vi "Delete.vi"() -> ()   [LabVIEW 2020]
uses:
  <vilib>/httpClient/LabVIEWHTTPClient.lvlib
panel:
  out "error out":errorcluster
  out "body":string
  out "headers":string
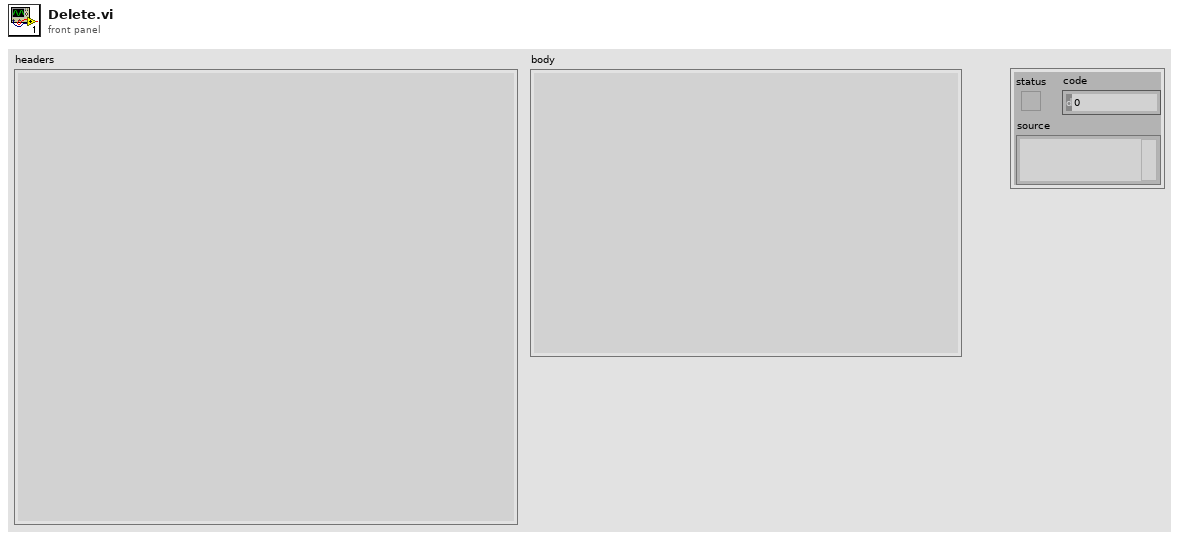
[diagram p1: front panel]
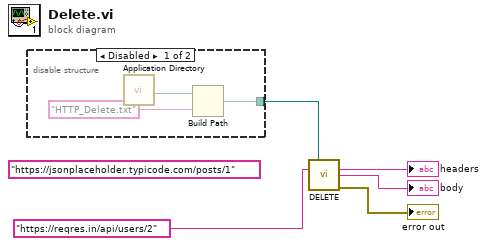
[diagram p0: block diagram]
diagram:
  (unwired) "https://jsonplaceholder.typicode.com/posts/1" ("url")
  n1 = disable-structure shown="Disabled" {
    disable-tunnel: [w6 _] -> w4
    frame Disabled {
      n2 = call <vilib>:"Application Directory.vi"() -> ("Application Directory"=w8:path)
      n3 = Build Path(base path=w8, name or relative path="HTTP_Delete.txt") -> (appended path=w6:path)
    }
    frame Enabled {
    }
  }
  n4 = call <vilib>:"DELETE.vi"("output file"=w4, "url"="https://reqres.in/api/users/2") -> ("headers"=→"headers":string, "body"=→"body":string, "error out"=→"error out":errorcluster)  [unwired: 10 in, 1 out]
